vi "Add Component.vi"(8 "error in (no error)":errorcluster, 9 "Qty":i32, 10 "Item":refnum<class "Item.lvclass">, 11 "Blueprint in":refnum<class "Blueprint.lvclass">) -> (0 "error out":errorcluster, 3 "Blueprint out":refnum<class "Blueprint.lvclass">)   [LabVIEW 2020, in "Blueprint.lvclass"]
uses:
  Blueprint.lvclass
  Item/Item.lvclass
  Item/Ingredient.ctl
  Blueprint.lvclass/Blueprint.ctl
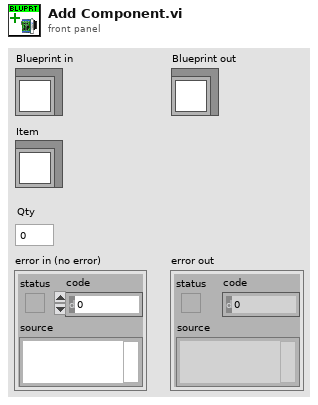
[diagram p1: front panel]
types:
  T1 = typedef "Item.lvclass/Ingredient.ctl" = cluster{"Item":refnum<class "Item.lvclass">, "Qty":dbl}
  T2 = typedef "Blueprint.lvclass/Ref Data.ctl" = cluster{"Ingredients":T1[], "Workstation":refnum<class "Workstation.lvclass">, "Craft Time":dbl, "Name":string}
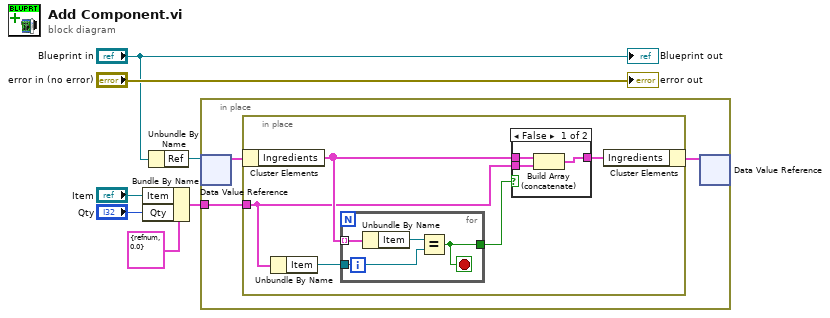
[diagram p0: block diagram]
diagram:
  n1 = Bundle By Name(cluster=T1 {"Item"=refnum, "Qty"=0.0} ("Ingredient"), "Item"="Item", "Qty"="Qty") -> (w1:T1)
  n2 = Unbundle By Name("Blueprint in") -> ("Ref"=w6:refnum<data-value>)
  n3 = in-place {
    in-place-border: w1 -> [w8]
    n4 = in-place-dvr #1(w6) -> (w10:T2)  [unwired: 1 out]
    n5 = in-place {
      in-place-border: w8 -> [w12]
      n6 = in-place-cluster #2(w10) -> ("Ingredients"=w13:T1[])
      n7 = Unbundle By Name(w12) -> ("Item"=w15:refnum<class "Item.lvclass">)
      n8 = for {
        tunnel: w13 -> [w23] mode=indexing
        tunnel: w15 -> [w21]
        tunnel: [w20] -> w14
        stop <- w20 stop-if-true
        n9 = Unbundle By Name(w23) -> ("Item"=w22:refnum<class "Item.lvclass">)
        n10 = Equal?(x=w22, y=w21) -> (x = y?=w20:bool)
      }
      n11 = case shown="False" w14 {
        tunnel: w13 -> [w18 w19]
        tunnel: w12 -> [w17 _]
        tunnel: [w16 w19] -> w11
        frame False {
          n12 = Build Array (concatenate)(w18, w17) -> (w16:T1[])
        }
        frame True {
        }
      }
      n13 = in-place-cluster #2("Ingredients"=w11) -> (w9:T2)
    }
    n14 = in-place-dvr #1(w9) -> ()  [unwired: 2 out]
  }
  "error out" <- "error in (no error)"
  "Blueprint out" <- "Blueprint in"
